vi "Remove.vi"(8 "error in (no error)":errorcluster, 11 "3D Object in":refnum<class "3D Object.lvclass">) -> (0 "error out":errorcluster)   [LabVIEW 2015, in "3D Object.lvclass"]
uses:
  3D Object.lvclass
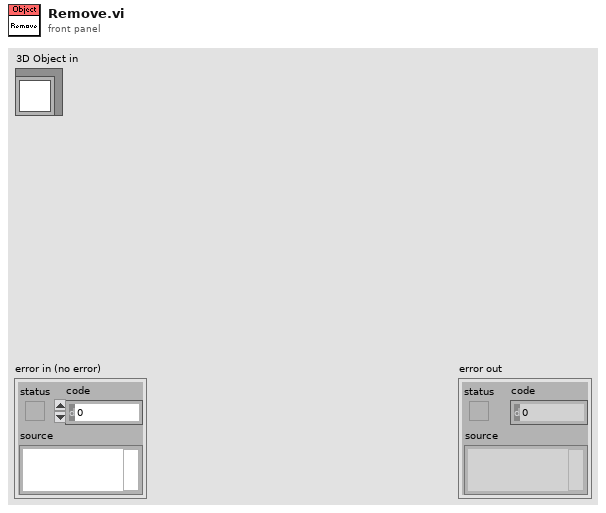
[diagram p1: front panel]
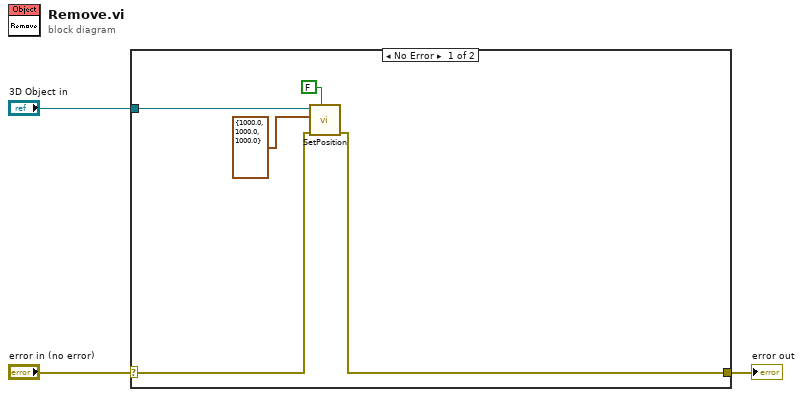
[diagram p0: block diagram]
diagram:
  n1 = case shown="No Error" "error in (no error)" {
    selector: "error in (no error)" -> [w4 w9]
    tunnel: [w5 w9] -> w2
    tunnel: "3D Object in" -> [w8 _]
    frame No Error {
      n2 = call "SetPosition.vi"("Relative?"=FALSE, "error in (no error)"=w4, "Position"=cluster{"X":sgl, "Y":sgl, "Z":sgl} {"X"=1000.0, "Y"=1000.0, "Z"=1000.0}, "3D Object in"=w8) -> ("error out"=w5:errorcluster)  [unwired: 6 in, 1 out]
    }
    frame Error {
    }
  }
  "error out" <- w2
